vi "InsertChData.vi"(8 "error in":errorcluster, 11 "检测数据":T1) -> (0 "error out":errorcluster)   [LabVIEW 2014, in "DataBase.lvlib"]
uses:
  DataBase.lvlib
  <vilib>/addons/database/Connection.llb/DB Tools Open Connec (String).vi
  <vilib>/addons/database/Connection.llb/Conn Execute.vi
  <vilib>/addons/database/Recordset.llb/Rec Destroy - Connection.vi
  <vilib>/addons/database/NI_Database_API.lvlib
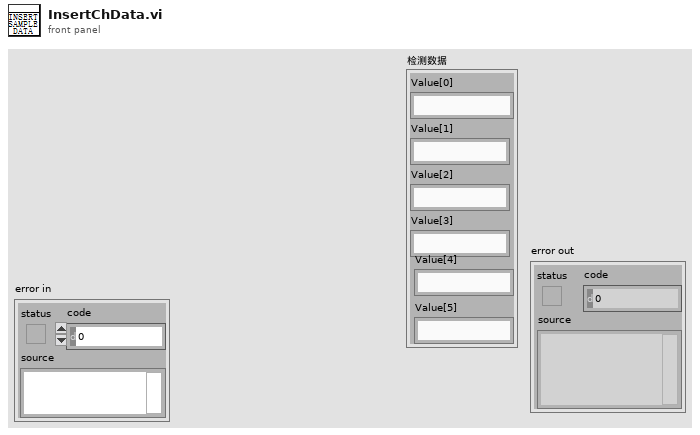
[diagram p1: front panel]
types:
  T1 = cluster{"Value[0]":string, "Value[1]":string, "Value[2]":string, "Value[3]":string, "Value[4]":string, "Value[5]":string}
  T2 = typedef "NI_Database_API.lvlib/Conn ObjectReference.ctl" = refnum<k1>
  T3 = typedef "NI_Database_API.lvlib/Rec ObjectReference.ctl" = refnum<k1>
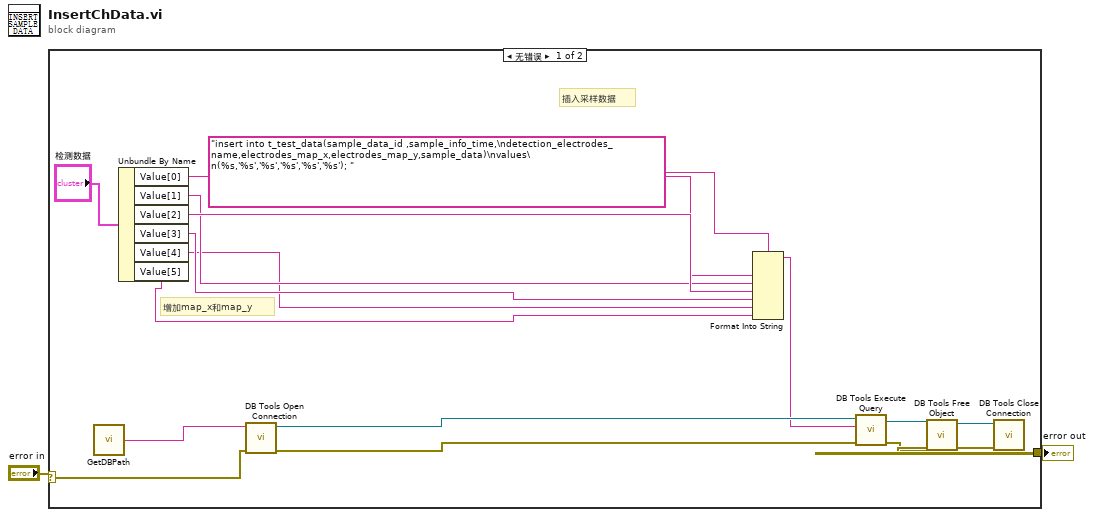
[diagram p0: block diagram]
diagram:
  n1 = case shown="无错误" "error in" {
    selector: "error in" -> [w16 w21]
    tunnel: [w15 w21] -> w1
    frame No Error {
      # "增加map_x和map_y"
      # "插入采样数据"
      n2 = call "GetDBPath.vi"() -> ("Connection"=w14:string)  [unwired: 1 in]
      n3 = Unbundle By Name("检测数据") -> ("Value[0]"=w9:string, "Value[1]"=w10:string, "Value[2]"=w11:string, "Value[3]"=w5:string, "Value[4]"=w4:string, "Value[5]"=w3:string)
      n4 = call-poly <vilib>:"DB Tools Open Connection.vi"("error in (no error)"=w16, "connection information"=w14) -> ("error out"=w19:errorcluster, "connection reference"=w20:T2)  [unwired: 6 in]
      n5 = Format Into String(format string="insert into t_test_data(sample_data_id ,sample_info_time,\ndetection_electrodes_name,electrodes_map_x,electrodes_map_y,sample_data)\nvalues\n(%s,'%s','%s','%s','%s','%s'); ", w9, w10, w11, w5, w4, w3) -> (resulting string=w6:string)  [unwired: 2 in, 1 out]
      n6 = call-poly <vilib>:"DB Tools Execute Query.vi"("error in (no error)"=w19, "SQL query"=w6, "connection reference"=w20) -> ("error out"=w12:errorcluster, "recordset reference"=w13:T3)  [unwired: 5 in]
      n7 = call-poly <vilib>:"DB Tools Free Object.vi"("error in (no error)"=w12, "recordset reference"=w13) -> ("error out"=w18:errorcluster, "connection reference"=w17:T2)  [unwired: 8 in]
      n8 = call <vilib>:"DB Tools Close Connection.vi"("error in (no error)"=w18, "connection reference"=w17) -> ("error out"=w15:errorcluster)  [unwired: 5 in]
    }
    frame Error {
    }
  }
  "error out" <- w1
